vi "Run Bfr Rx - Handle Data.vi"(7 "Buffer Option Support in":T1 {"Ping Pong Buffer"."Active Buffer Ref" format="%016x"; "Cached Buffer"."Cache Buffer" format="%016x"}, 8 "error in (no error)":errorcluster, 10 "Data":u8[](array[numeric]), 11 "Buffer Resources":T7 {"Data Buffer" format="%016x"}) -> (0 "error out":errorcluster, 4 "Data Size":u64, 5 "Buffer Option Support out":T1 {"Ping Pong Buffer"."Active Buffer Ref" format="%016x"; "Cached Buffer"."Cache Buffer" format="%016x"})   [LabVIEW 2021, in "UDP-Custom-Device Engine.lvlib"]
uses:
  UDP-Custom-Device Engine.lvlib
  Types/Engine - Buffer Resources.ctl
  Shared/Types/Shared - Pointer Encoding.ctl
  Types/Engine - Buffered Rx Buffer Option Support.ctl
  Shared/Types/Shared - Receive Buffer Options.ctl
  Types/Engine - Buffered Rx Circular Buffer.ctl
  Types/Engine - Buffered Rx Cached Buffer.ctl
  Types/Engine - Buffered Rx Ping Pong Buffer.ctl
  Types/Engine - Buffered Rx Active Buffer.ctl
  <vilib>/NI VeriStand/VeriStand Data/Pointer Operations/Pointer.Write (1D U8).vi
  <vilib>/NI VeriStand/VeriStand Data/Pointer Operations/Pointer.Write (I32).vi
  Block Cache and Size/Run Bfr Rx - Cached - Copy Cache.vi
  Block Cache and Size/Run Bfr Rx - Cached - Flush Cache.vi
  Block Cache and Size/Run Bfr Rx - Cached - Add to Cache.vi
  Block Cache and Size/Run Bfr Rx - CachedSize - Copy Cache.vi
  Block Cache and Size/Run Bfr Rx - CachedSize - Flush Cache.vi
  Block Cache and Size/Run Bfr Rx - CachedSize - Add to Cache.vi
  Ping Pong and Size/Run Bfr Rx - PingPong - Change Buffer.vi
  Ping Pong and Size/Run Bfr Rx - PingPong - Flush Active.vi
  Ping Pong and Size/Run Bfr Rx - PingPong - Add to Active.vi
  Ping Pong and Size/Run Bfr Rx - PingPongSized - Change Buffer.vi
  Ping Pong and Size/Run Bfr Rx - PingPongSized - Flush Active.vi
  Ping Pong and Size/Run Bfr Rx - PingPongSized - Add to Active.vi
  <vilib>/NI VeriStand/VeriStand Data/Pointer Operations/Pointer.In-Place Read.vi
  <vilib>/NI VeriStand/VeriStand Data/Pointer Operations/Pointer.In-Place Read (1D U8).vi
  <vilib>/NI VeriStand/VeriStand Data/Pointer Operations/Pointer.Read (U16).vi
  <vilib>/NI VeriStand/VeriStand Data/Pointer Operations/Pointer.Write (U16).vi
  <vilib>/NI VeriStand/VeriStand Data/Pointer Operations/Pointer.Write (U8).vi
  <vilib>/NI VeriStand/VeriStand Data/Pointer Operations/Pointer.In-Place Read (U16).vi
  <vilib>/NI VeriStand/VeriStand Data/VeriStand Data.lvlib
  <vilib>/NI VeriStand/VeriStand Data/Pointer Operations/Pointer.Read (1D U8).vi
  Shared/UDP-Custom-Device Shared.lvlib
panel:
  out "copyFlush":bool
  out "cache":string
  out "buffer":string
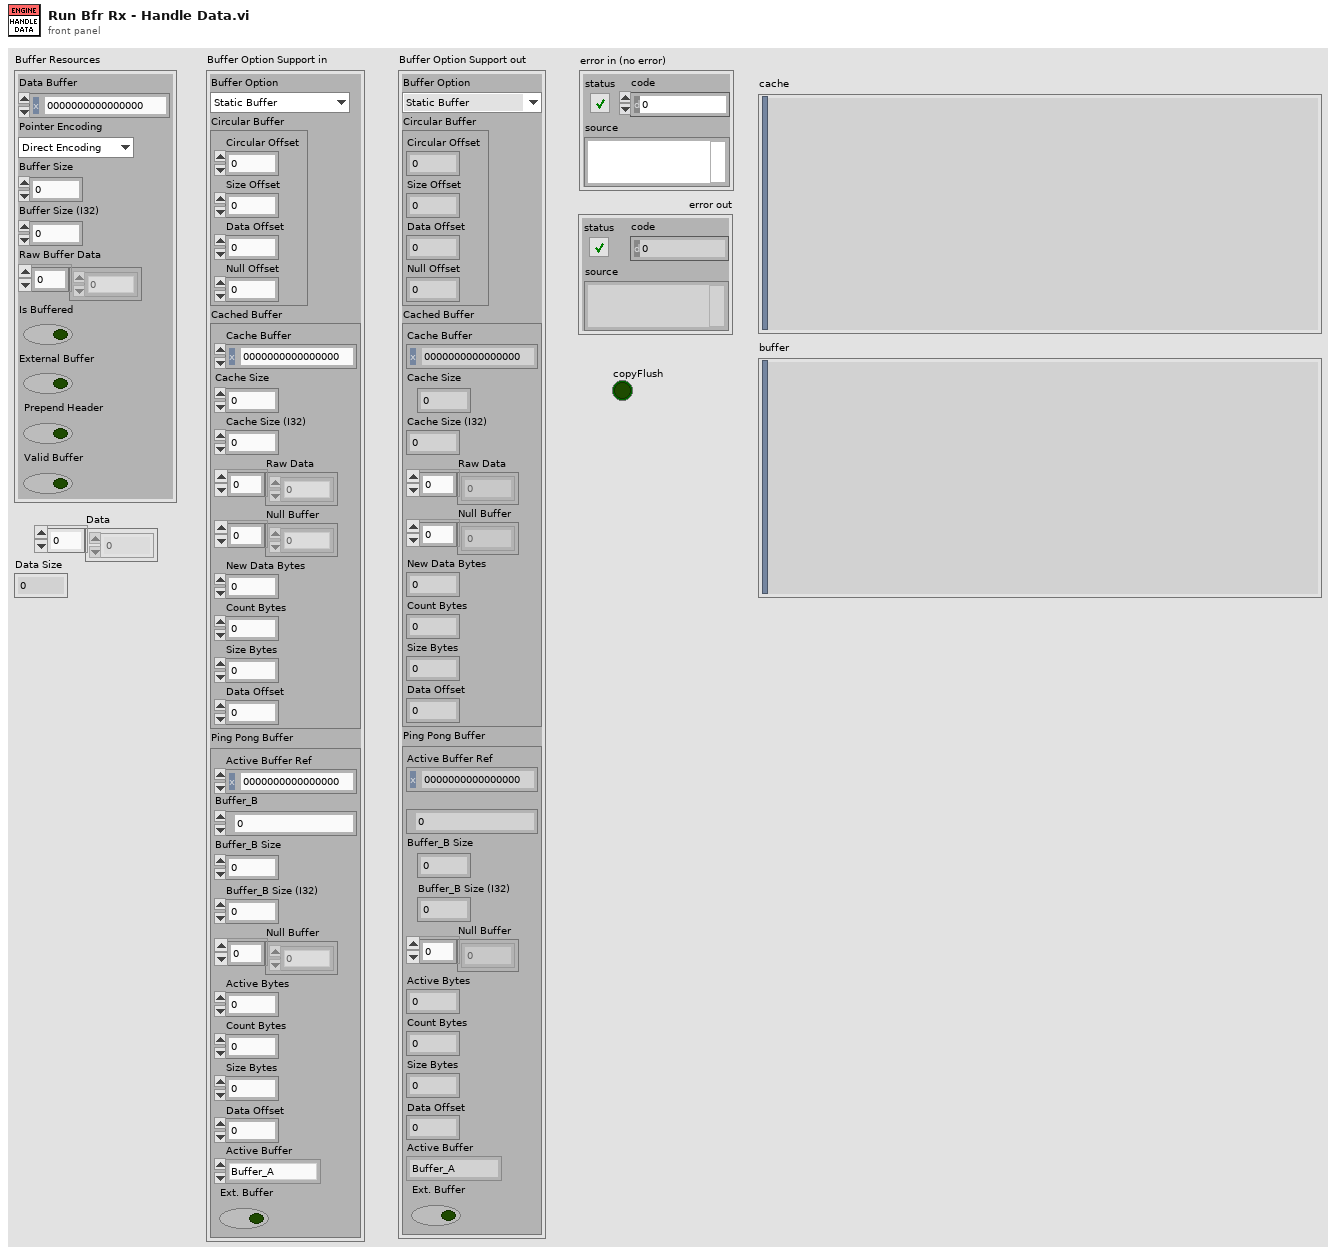
[diagram p1: front panel]
types:
  T1 = typedef "UDP-Custom-Device Engine.lvlib/Engine - Buffered Rx Buffer Option Support.ctl" = cluster{"Buffer Option":T2, "Circular Buffer":T3, "Cached Buffer":T4, "Ping Pong Buffer":T5}
  T2 = typedef "UDP-Custom-Device Shared.lvlib/Shared - Receive Buffer Options.ctl" = enum16{"Static Buffer", "Circular Buffer", "Circular Buffer + Size", "Internal Cache", "Internal Cache + Size", "Ping Pong", "Ping Pong + Size"}
  T3 = typedef "UDP-Custom-Device Engine.lvlib/Engine - Buffered Rx Circular Buffer.ctl" = cluster{"Circular Offset":u64, "Size Offset":u64, "Data Offset":u64, "Null Offset":u64}
  T4 = typedef "UDP-Custom-Device Engine.lvlib/Engine - Buffered Rx Cached Buffer.ctl" = cluster{"Cache Buffer":u64, "Cache Size":u64, "Cache Size (I32)":i32, "Raw Data":u8[], "Null Buffer":u8[], "New Data Bytes":u64, "Count Bytes":u64, "Size Bytes":u64, "Data Offset":u64}
  T5 = typedef "UDP-Custom-Device Engine.lvlib/Engine - Buffered Rx Ping Pong Buffer.ctl" = cluster{"Active Buffer Ref":u64, "Buffer_B":u64, "Buffer_B Size":u64, "Buffer_B Size (I32)":i32, "Null Buffer":u8[], "Active Bytes":u64, "Count Bytes":u64, "Size Bytes":u64, "Data Offset":u64, "Active Buffer":T6, "Ext. Buffer":bool}
  T6 = typedef "UDP-Custom-Device Engine.lvlib/Engine - Buffered Rx Active Buffer.ctl" = enum16{"Buffer_A", "Buffer_B"}
  T7 = typedef "UDP-Custom-Device Engine.lvlib/Engine - Buffer Resources.ctl" = cluster{"Data Buffer":u64, "Pointer Encoding":T8, "Buffer Size":u64, "Buffer Size (I32)":i32, "Raw Buffer Data":u8[], "Is Buffered":bool, "External Buffer":bool, "Prepend Header":bool, "Valid Buffer":bool}
  T8 = typedef "UDP-Custom-Device Shared.lvlib/Shared - Pointer Encoding.ctl" = enum16{"Direct Encoding", "Conversion Encoding"}
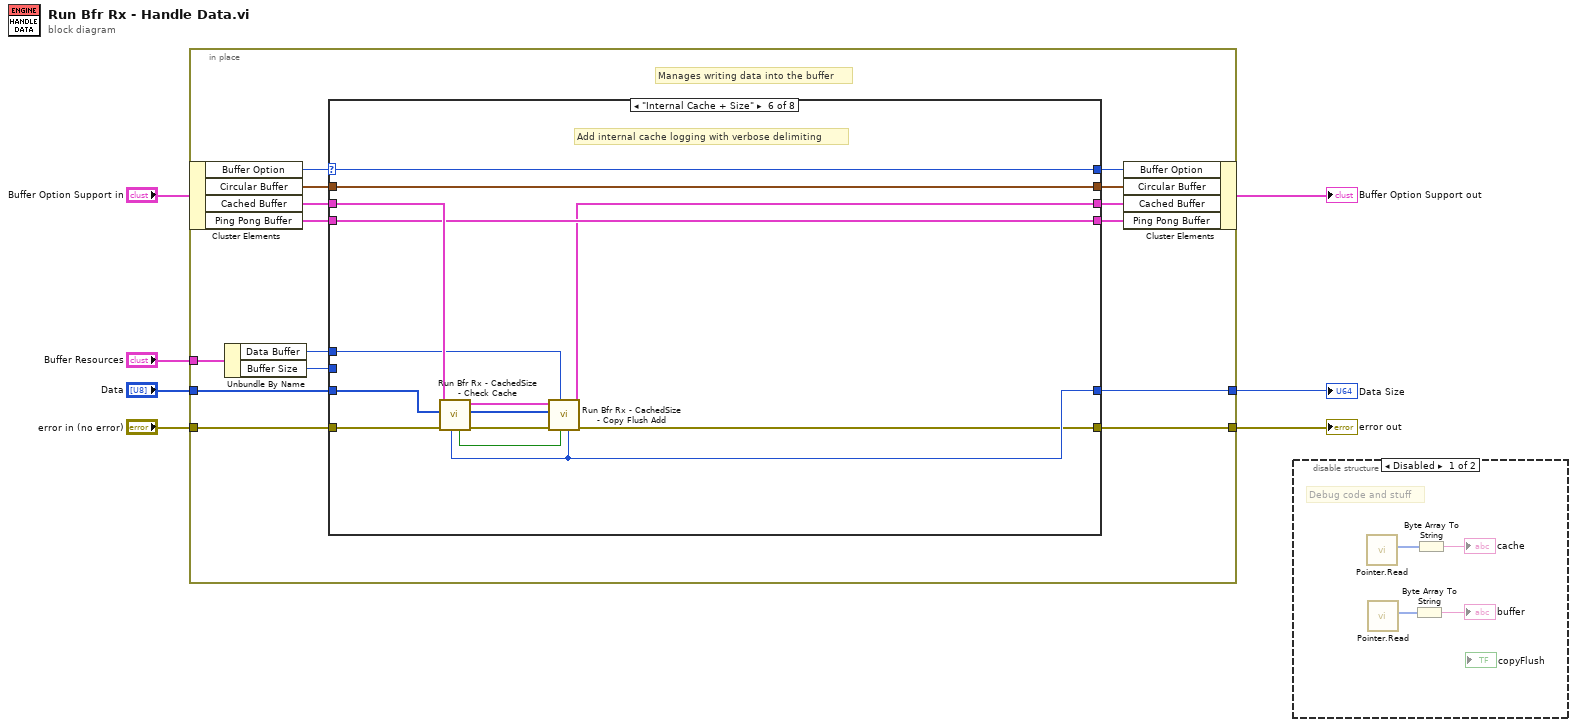
[diagram p0: block diagram]
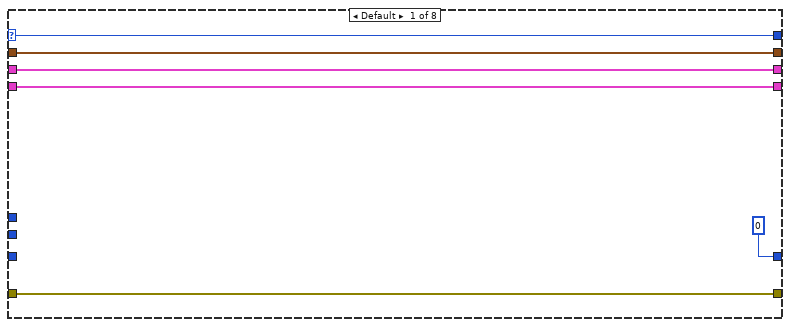
[diagram p3: hidden frame]
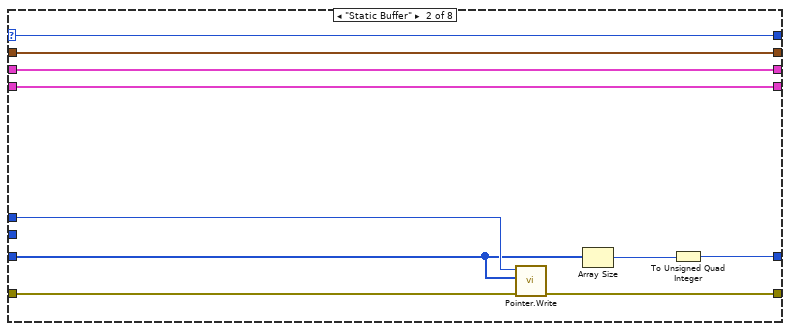
[diagram p4: hidden frame]
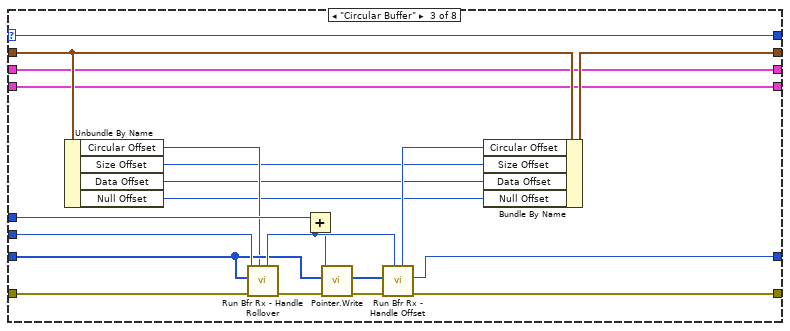
[diagram p5: hidden frame]
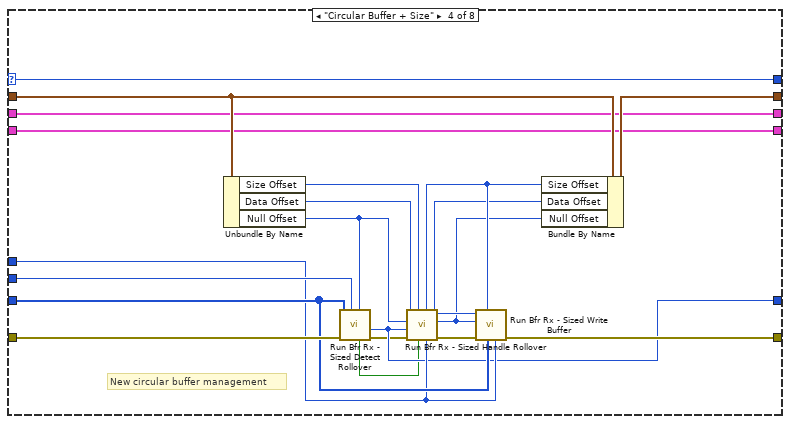
[diagram p6: hidden frame]
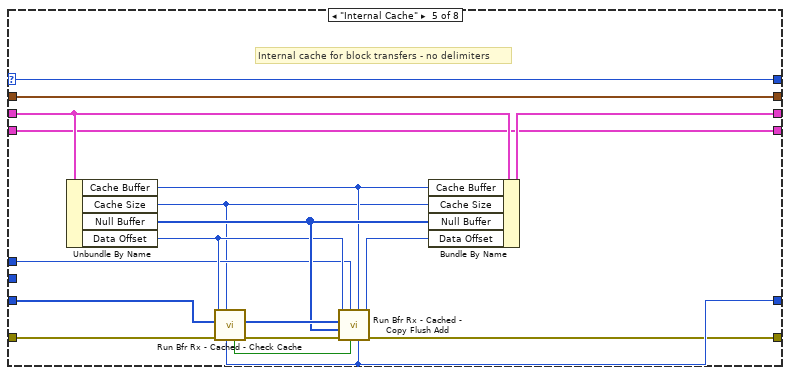
[diagram p7: hidden frame]
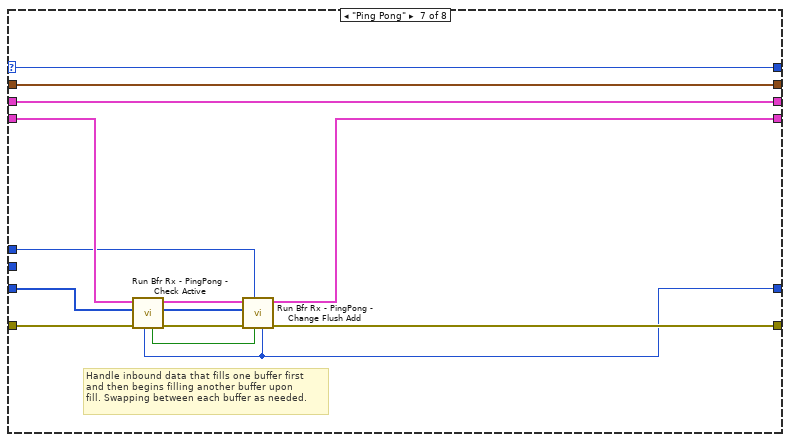
[diagram p8: hidden frame]
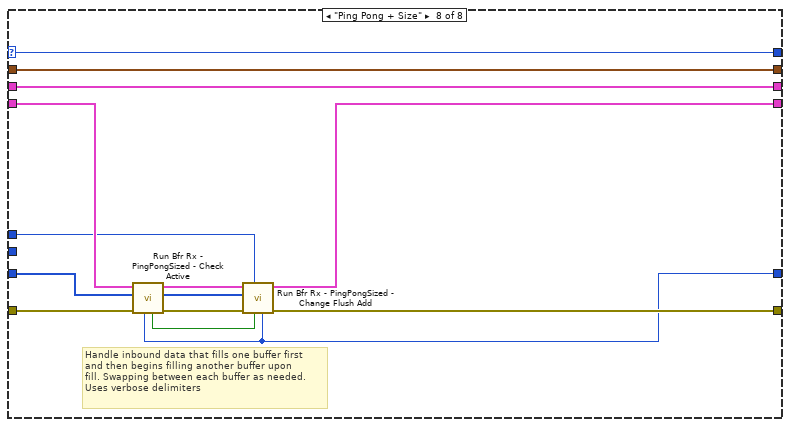
[diagram p9: hidden frame]
diagram:
  n1 = in-place {
    in-place-border: "Data" -> [w22]
    in-place-border: "error in (no error)" -> [w21]
    in-place-border: [w20] -> w5
    in-place-border: [w19] -> w4
    in-place-border: "Buffer Resources" -> [w18]
    # "Manages writing data into the buffer"
    n2 = in-place-cluster #1("Buffer Option Support in") -> ("Buffer Option"=w15:T2, "Circular Buffer"=w13:T3, "Cached Buffer"=w11:T4, "Ping Pong Buffer"=w8:T5)
    n3 = Unbundle By Name(w18) -> ("Data Buffer"=w17:u64, "Buffer Size"=w16:u64)
    n4 = case shown="\"Internal Cache + Size\"" w15 {
      selector: w15 -> [w26 w37 w53 w73 w97 w110 w123 w137]
      tunnel: w17 -> [_ w36 w55 w76 w83 w98 w113 w126]
      tunnel: w22 -> [_ w35 w51 w78 w95 w107 w122 w135]
      tunnel: w21 -> [w25 w34 w56 w79 w94 w108 w121 w134]
      tunnel: [w25 w33 w59 w75 w81 w102 w117 w132] -> w20
      tunnel: w16 -> [_ _ w54 w77 _ _ _ _]
      tunnel: [u64 0 ("Data Size (U64)") w30 w58 w74 w88 w103 w116 w131] -> w19
      tunnel: [w26 w37 w53 w73 w97 w110 w123 w137] -> w14
      tunnel: w13 -> [w28 w32 w46 w63 w96 w111 w125 w139]
      tunnel: [w28 w32 w45 w62 w96 w111 w125 w139] -> w12
      tunnel: w11 -> [w27 w31 w40 w61 w90 w109 w124 w138]
      tunnel: [w27 w31 w40 w61 w89 w99 w124 w138] -> w10
      tunnel: [w23 w29 w39 w60 w80 w101 w114 w127] -> w9
      tunnel: w8 -> [w23 w29 w39 w60 w80 w101 w119 w136]
      frame Default {
      }
      frame "Static Buffer" {
        n5 = call-poly <vilib>:"Pointer.Write.vi"("error in (no error)"=w34, "values"=w35, "pointer in"=w36) -> ("error out"=w33:errorcluster)  [unwired: 6 in, 2 out]
        n6 = Array Size(array=w35) -> (size(s)=w38:i32)
        n7 = To Unsigned Quad Integer(1:w38) -> (0:w30:u64)
      }
      frame "Circular Buffer" {
        n8 = Unbundle By Name(w46) -> ("Circular Offset"=w47:u64, "Size Offset"=w43:u64, "Data Offset"=w42:u64, "Null Offset"=w41:u64)
        n9 = call "Run Bfr Rx - Handle Rollover.vi"("Offset in"=w47, "error in (no error)"=w56, "Data in"=w51, "Buffer Size"=w54) -> ("error out"=w48:errorcluster, "Offset out"=w57:u64)  [unwired: 5 in, 1 out]
        n10 = Add(x=w55, y=w57) -> (x+y=w52:u64)
        n11 = call-poly <vilib>:"Pointer.Write.vi"("error in (no error)"=w48, "values"=w51, "pointer in"=w52) -> ("error out"=w49:errorcluster, "values out"=w50:u8[])  [unwired: 6 in, 1 out]
        n12 = call "Run Bfr Rx - Handle Offset.vi"("Offset in"=w57, "error in (no error)"=w49, "Data"=w50) -> ("error out"=w59:errorcluster, "Data Size"=w58:u64, "Offset out"=w44:u64)  [unwired: 5 in, 1 out]
        n13 = Bundle By Name(cluster=w46, "Circular Offset"=w44, "Size Offset"=w43, "Data Offset"=w42, "Null Offset"=w41) -> (w45:T3)
      }
      frame "Circular Buffer + Size" {
        # "New circular buffer management"
        n14 = Unbundle By Name(w63) -> ("Size Offset"=w67:u64, "Data Offset"=w68:u64, "Null Offset"=w69:u64)
        n15 = call "Run Bfr Rx - Sized Detect Rollover.vi"("Null Offset"=w69, "Buffer Size"=w77, "error in (no error)"=w79, "Data"=w78) -> ("error out"=w72:errorcluster, "Data Size (U64)"=w74:u64, "Rollover Occurred?"=w71:bool)  [unwired: 5 in]
        n16 = call "Run Bfr Rx - Sized Handle Rollover.vi"("Data Buffer"=w76, "Rollover Occurred?"=w71, "Size Offset in"=w67, "error in (no error)"=w72, "Data Size (I32)"=w74, "Null Offset in"=w69, "Data Offset in"=w68) -> ("error out"=w70:errorcluster, "Null Offset out"=w64:u64, "Data Offset out"=w65:u64, "Size Offset out"=w66:u64)  [unwired: 1 in]
        n17 = call "Run Bfr Rx - Sized Write Buffer.vi"("Data Buffer"=w76, "Data"=w78, "Size Offset in"=w66, "error in (no error)"=w70, "Null Offset in"=w64, "Data Offset in"=w65) -> ("error out"=w75:errorcluster)  [unwired: 5 in]
        n18 = Bundle By Name(cluster=w63, "Size Offset"=w66, "Data Offset"=w65, "Null Offset"=w64) -> (w62:T3)
      }
      frame "Internal Cache" {
        # "Internal cache for block transfers - no delimiters"
        n19 = Unbundle By Name(w90) -> ("Cache Buffer"=w84:u64, "Cache Size"=w82:u64, "Null Buffer"=w86:u8[], "Data Offset"=w85:u64)
        n20 = call "Run Bfr Rx - Cached - Check Cache.vi"("Cache Size"=w82, "error in (no error)"=w94, "Data in"=w95, "Data Offset in"=w85) -> ("error out"=w92:errorcluster, "Data out"=w93:u8[], "Copy and Flush"=w87:bool, "Data Size out"=w88:u64)  [unwired: 4 in]
        n21 = call "Run Bfr Rx - Cached - Copy Flush Add.vi"("Data Size in"=w88, "Cache Buffer"=w84, "Copy and Flush"=w87, "External Buffer"=w83, "error in (no error)"=w92, "Null Data in"=w86, "Data in"=w93, "Data Offset in"=w85) -> ("error out"=w81:errorcluster, "Data Offset out"=w91:u64)  [unwired: 2 in]
        n22 = Bundle By Name(cluster=w90, "Cache Buffer"=w84, "Cache Size"=w82, "Null Buffer"=w86, "Data Offset"=w91) -> (w89:T4)
      }
      frame "Internal Cache + Size" {
        # "Add internal cache logging with verbose delimiting"
        n23 = call "Run Bfr Rx - CachedSize - Check Cache.vi"("error in (no error)"=w108, "Data in"=w107, "Cached Buffer in"=w109) -> ("error out"=w105:errorcluster, "Data out"=w104:u8[], "Cached Buffer out"=w106:T4, "Copy and Flush"=w100:bool, "Data Size out"=w103:u64)  [unwired: 4 in]
        n24 = call "Run Bfr Rx - CachedSize - Copy Flush Add.vi"("Data Size in"=w103, "Copy and Flush"=w100, "External Buffer"=w98, "error in (no error)"=w105, "Data in"=w104, "Cached Buffer in"=w106) -> ("error out"=w102:errorcluster, "Cached Buffer out"=w99:T4)  [unwired: 4 in]
      }
      frame "Ping Pong" {
        # "Handle inbound data that fills one buffer first\nand then begins filling another buffer upon\nfill. Swapping between each buffer as needed."
        n25 = call "Run Bfr Rx - PingPong - Check Active.vi"("error in (no error)"=w121, "Data in"=w122, "Ping Pong Buffer in"=w119) -> ("error out"=w118:errorcluster, "Data out"=w115:u8[], "Ping Pong Buffer out"=w120:T5, "Change Active"=w112:bool, "Data Size out"=w116:u64)  [unwired: 4 in]
        n26 = call "Run Bfr Rx - PingPong - Change Flush Add.vi"("Data Size in"=w116, "Change Active"=w112, "Buffer_A"=w113, "error in (no error)"=w118, "Data in"=w115, "Ping Pong Buffer in"=w120) -> ("error out"=w117:errorcluster, "Ping Pong Buffer out"=w114:T5)  [unwired: 4 in]
      }
      frame "Ping Pong + Size" {
        # "Handle inbound data that fills one buffer first\nand then begins filling another buffer upon\nfill. Swapping between each buffer as needed.\nUses verbose delimiters"
        n27 = call "Run Bfr Rx - PingPongSized - Check Active.vi"("error in (no error)"=w134, "Data in"=w135, "Ping Pong Buffer in"=w136) -> ("error out"=w130:errorcluster, "Data out"=w129:u8[], "Ping Pong Buffer out"=w133:T5, "Change Active"=w128:bool, "Data Size out"=w131:u64)  [unwired: 4 in]
        n28 = call "Run Bfr Rx - PingPongSized - Change Flush Add.vi"("Data Size in"=w131, "Change Active"=w128, "Buffer_A"=w126, "error in (no error)"=w130, "Data in"=w129, "Ping Pong Buffer in"=w133) -> ("error out"=w132:errorcluster, "Ping Pong Buffer out"=w127:T5)  [unwired: 4 in]
      }
    }
    n29 = in-place-cluster #1("Buffer Option"=w14, "Circular Buffer"=w12, "Cached Buffer"=w10, "Ping Pong Buffer"=w9) -> (→"Buffer Option Support out":T1)
  }
  "error out" <- w5
  "Data Size" <- w4
  n30 = disable-structure shown="Disabled" {
    frame Disabled {
      # "Debug code and stuff"
      n31 = call-poly <vilib>:"Pointer.Read.vi"() -> ("values"=w142:u8[])  [unwired: 9 in, 2 out]
      n32 = call-poly <vilib>:"Pointer.Read.vi"() -> ("values"=w143:u8[])  [unwired: 9 in, 2 out]
      n33 = Byte Array To String(unsigned byte array=w143) -> (string=→"buffer":string)
      n34 = Byte Array To String(unsigned byte array=w142) -> (string=→"cache":string)
    }
    frame Enabled {
    }
  }
